vi "Set Control Data.vi"(7 "UID":i32, 8 "error in (no error)":errorcluster, 10 "Value":string, 11 "Web FP In":refnum<class "Web Front Panel.lvclass">) -> (0 "error out":errorcluster, 3 "Web FP Out":refnum<class "Web Front Panel.lvclass">)   [LabVIEW 2017, in "Front Panel Publisher.lvlib" / "Web Front Panel.lvclass"]
uses:
  Web Front Panel.lvclass
  Front Panel Objects/Object_class/Object.lvclass
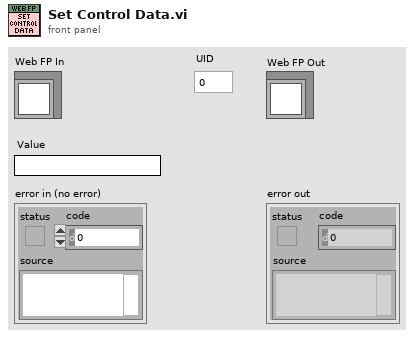
[diagram p1: front panel]
types:
  T1 = typedef "Front Panel Publisher.lvlib/Web Front Panel.lvclass/Object Attributes.ctl" = cluster{"VI Identifier":string, "VI Reference":refnum<vi>, "Controls":refnum<class "Object.lvclass">[], "Indicators":refnum<class "Object.lvclass">[], "Decorations":refnum<class "Object.lvclass">[], "VR With Previous Get":refnum<data-value>, "VR With Ring Images":refnum<data-value>}
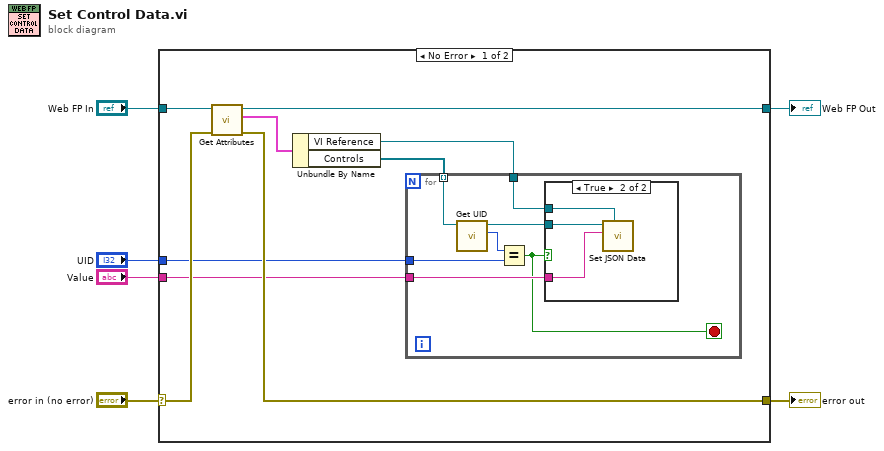
[diagram p0: block diagram]
diagram:
  n1 = case shown="No Error" "error in (no error)" {
    selector: "error in (no error)" -> [w15 w27]
    tunnel: [w13 w27] -> w5
    tunnel: [w11 w26] -> w3
    tunnel: "Web FP In" -> [w12 w26]
    tunnel: "UID" -> [w9 _]
    tunnel: "Value" -> [w7 _]
    frame No Error {
      n2 = call "Get Attributes.vi"("error in (no error)"=w15, "Web FP In"=w12) -> ("error out"=w13:errorcluster, "Data"=w14:T1, "Web FP Out"=w11:refnum<class "Web Front Panel.lvclass">)  [unwired: 6 in, 1 out]
      n3 = Unbundle By Name(w14) -> ("VI Reference"=w8:refnum<vi>, "Controls"=w10:refnum<class "Object.lvclass">[])
      n4 = for {
        tunnel: w10 -> [w22] mode=indexing
        tunnel: w9 -> [w20]
        tunnel: w8 -> [w18]
        tunnel: w7 -> [w17]
        stop <- w16 stop-if-true
        n5 = call-dynamic "Get UID.vi"("Object In"=w22) -> ("UID"=w21:i32, "Object In"=w19:refnum<class "Object.lvclass">)  [unwired: 8 in, 1 out]
        n6 = Equal?(x=w21, y=w20) -> (x = y?=w16:bool)
        n7 = case shown="True" w16 {
          tunnel: w19 -> [_ w25]
          tunnel: w18 -> [_ w24]
          tunnel: w17 -> [_ w23]
          frame False {
          }
          frame True {
            n8 = call-dynamic "Set JSON Data.vi"("VI Reference"=w24, "Value"=w23, "Object In"=w25) -> ()  [unwired: 7 in, 2 out]
          }
        }
      }
    }
    frame Error {
    }
  }
  "error out" <- w5
  "Web FP Out" <- w3
